vi "Timer.vi"(8 "error in (no error)":errorcluster, 9 "Pause":bool, 10 "Reset":bool, 11 "Target Time":dbl) -> (0 "error out":errorcluster, 2 "Elapsed?":bool, 3 "Elapsed TIme":dbl)   [LabVIEW 2013]
doc: "This subVI has following funcnality\n1.Pause- When it is pressed it stops the running elapsed time to the current value.\n2.Reset- Change the elapsed time value to zero.\n3.Elapsed; On- Time is elapsed\n Off- Time has not elapsed.\n4.Elapsed Time- Count the elapsed time"
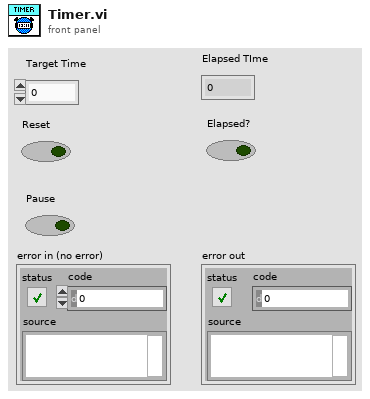
[diagram p1: front panel]
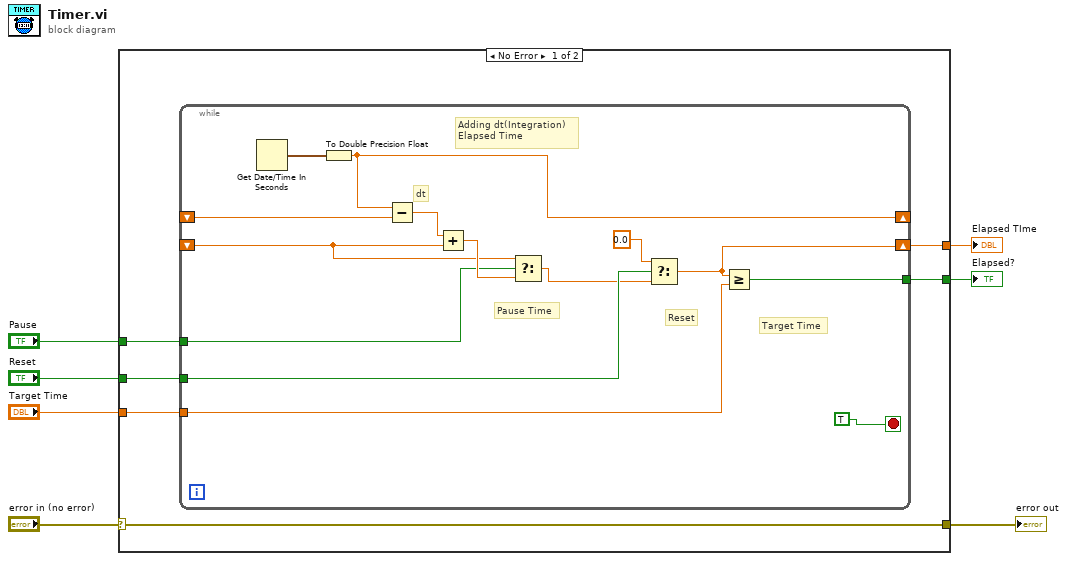
[diagram p0: block diagram]
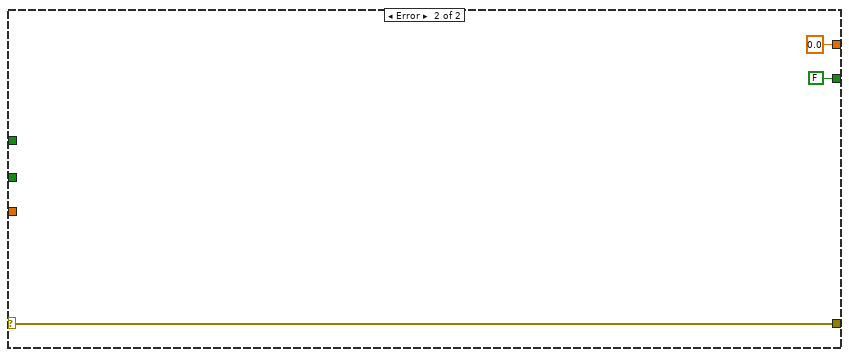
[diagram p2: hidden frame]
diagram:
  n1 = case shown="No Error" "error in (no error)" {
    selector: "error in (no error)" -> [w8 w30]
    tunnel: [w13 0.0 ("t")] -> w1
    tunnel: "Target Time" -> [w12 _]
    tunnel: [w11 FALSE] -> w3
    tunnel: "Reset" -> [w10 _]
    tunnel: "Pause" -> [w9 _]
    tunnel: [w8 w30] -> w7
    frame No Error {
      n2 = while {
        shift-right: [w25] -> _
        shift-left: _ -> [w26]
        shift-right: [w19] -> w13
        shift-left: _ -> [w16]
        tunnel: w12 -> [w23]
        tunnel: [w22] -> w11
        tunnel: w10 -> [w20]
        tunnel: w9 -> [w14]
        stop <- TRUE stop-if-true
        # "Target Time"
        # "Reset"
        # "Pause Time"
        # "Adding dt(Integration)\nElapsed Time"
        # "dt"
        n3 = Get Date/Time In Seconds() -> (seconds since 1Jan1904=w27:timestamp)
        n4 = To Double Precision Float(number=w27) -> (double precision float=w25:dbl)
        n5 = Subtract(x=w25, y=w26) -> (x-y=w24:dbl)
        n6 = Add(x=w24, y=w16) -> (x+y=w17:dbl)
        n7 = Select(t=w16, s=w14, f=w17) -> (s? t:f=w15:dbl)
        n8 = Select(t=0.0, s=w20, f=w15) -> (s? t:f=w19:dbl)
        n9 = Greater Or Equal?(x=w19, y=w23) -> (x >= y?=w22:bool)
      }
    }
    frame Error {
    }
  }
  "error out" <- w7
  "Elapsed?" <- w3
  "Elapsed TIme" <- w1
